vi "Update Graphs_Brass.vi"(0 "Select Graph":T8=enum."Water Temperature (F)", 2 "appended array":refnum<vi>[](array[refnum]), 5 "ERD Graph  Ind 2":T7, 7 "All_Bundled_Data_Brass":T1, 11 "Error In":errorcluster) -> (3 "Dryer Loads":dbl[][](graph), 4 "Washer Loads":u16[][](graph)=[[0, 100, 200, 300, 400]], 6 "Water Temperature":dbl(graph), 8 "Basket Speed":u16(graph), 10 "Pressure":dbl(graph), 12 "ERD 3":dbl(graph), 13 "ERD 2":dbl(graph), 14 "ERD 1":dbl(graph), 15 "Error Out":errorcluster)   [LabVIEW 2016]
doc: "This VI displays (makes visable) the corresponding graph based on user selection, as well as updates the values of the graphs with current data."
uses:
  type defs2/Select _Graph_Brass.ctl
  type defs2/All_Bundled_Data_Brass.ctl
  Laundry Tool 1.0 Support/type defs/Version.ctl
  type defs2/ERD_Always_Show_Brass.ctl
  type defs2/CSV_File_String_Arrays.ctl
  type defs2/Fault Table Array.ctl
  Laundry Tool 1.0 Support/type defs/Fault_Table_Info.ctl
panel:
  # "Software Version"
  # "UI - Critical Version"
  # "UI - Non-Critical"
  # "MC -  Version"
  # "Inverter Version"
  # "Model Setting"
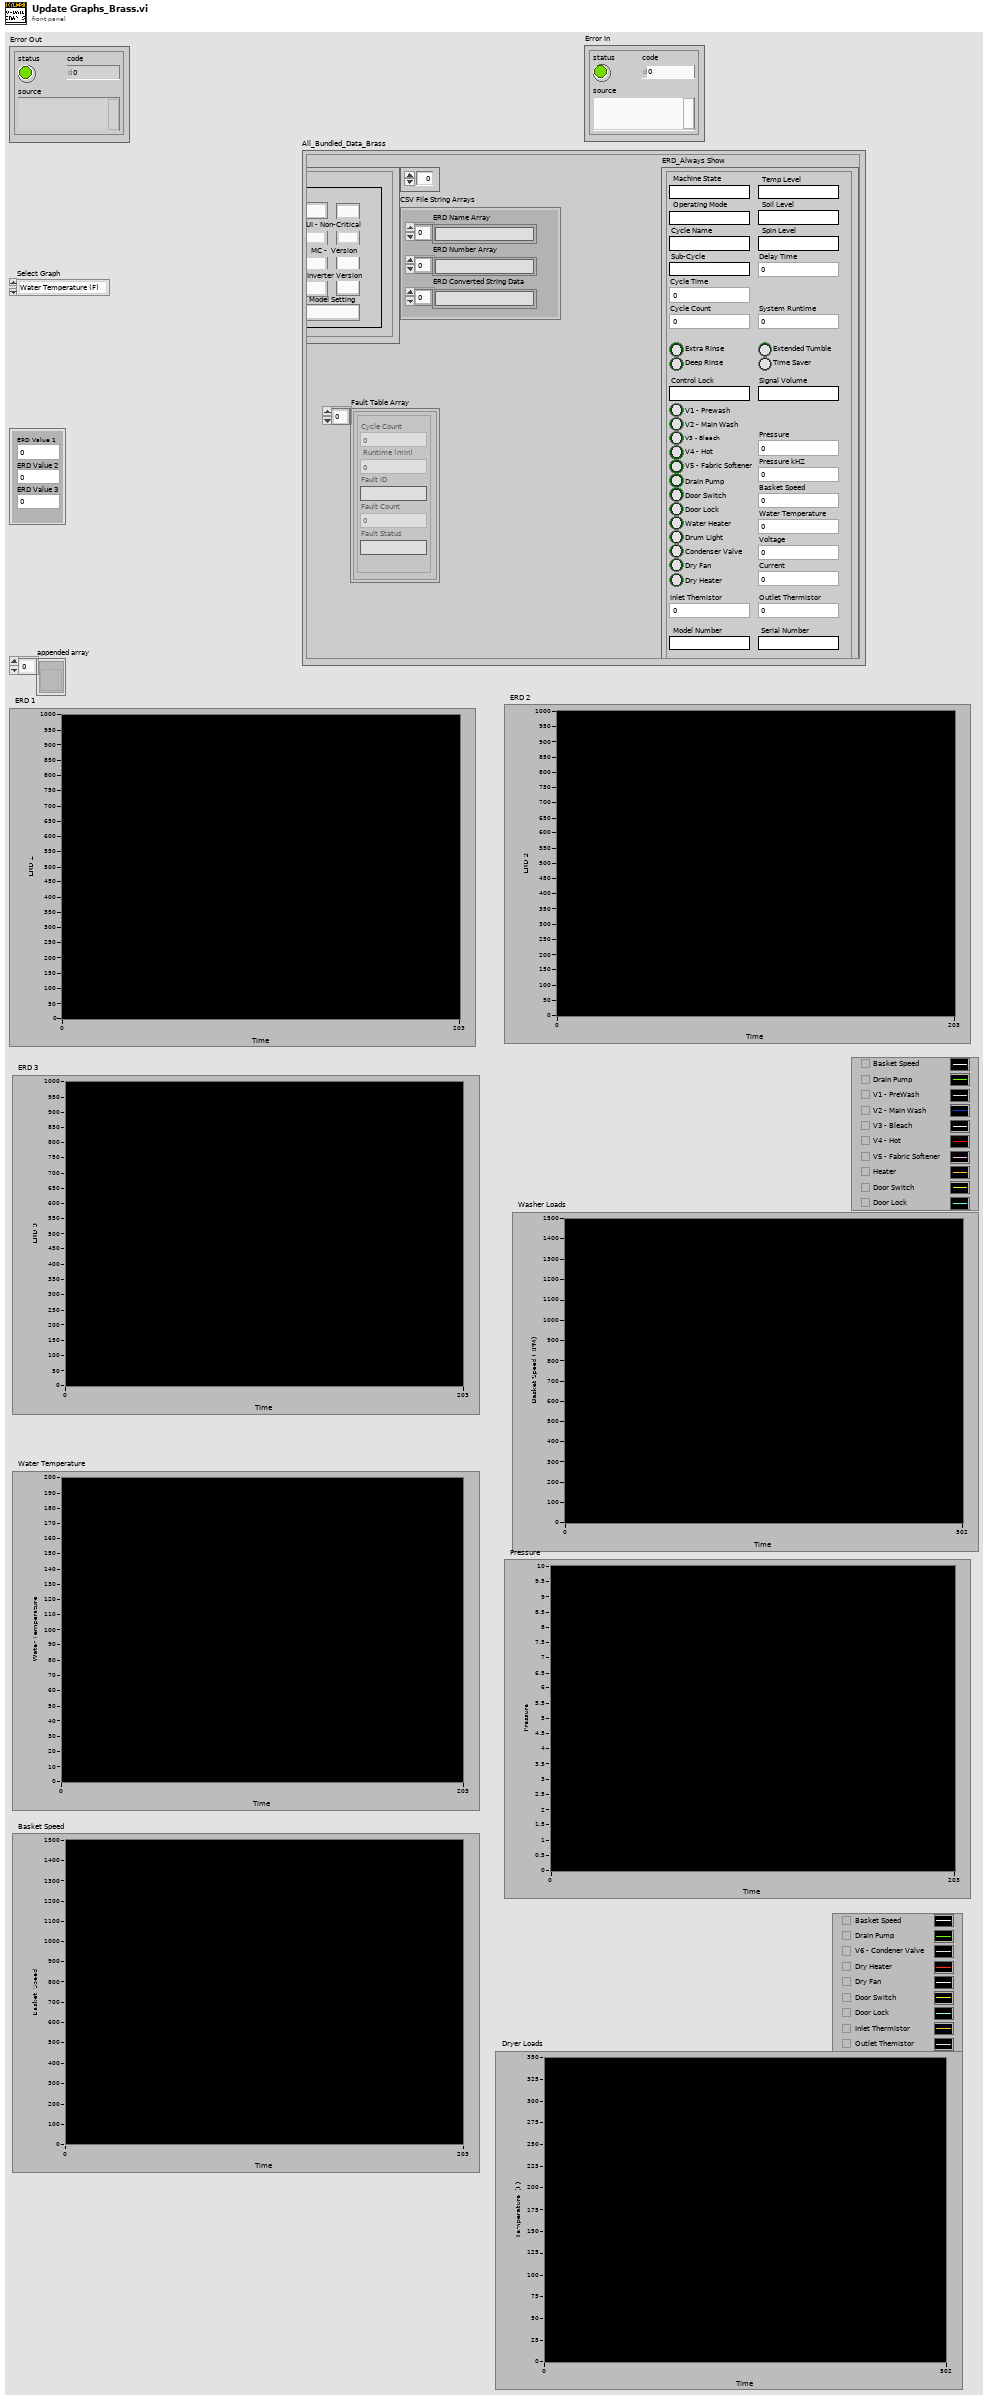
[diagram p1: front panel]
types:
  T1 = typedef "All_Bundled_Data_Brass.ctl" = cluster{"Version":T2, "ERD_Always Show":T3, "Personality Set":u8, "CSV File String Arrays":T4, "Fault Table Array ":T5}
  T2 = typedef "Version.ctl" = cluster{"UI - Critical Major":string, "UI - Critical Minor":string, "UI - Non-Critical Minor":string, "UI - Non-Critical Major":string, "MC Minor":string, "MC Major":string, "Model Setting":string, "Inverter Version  Minor":string, "Inverter Version Major":string}
  T3 = typedef "ERD_Always_Show_Brass.ctl" = cluster{"Machine State":string, "Cycle Count":u32, "Soil Level":string, "Spin Level":string, "Temp Level":string, "Delay Time":u16, "Sub-Cycle":string, "Cycle Name":string, "Model Number":string, "Serial Number":string, "System Runtime":u32, "Cycle Time":u16, "Operating Mode":string, "Deep Rinse":bool, "Extra Rinse":bool, "V1 - Prewash":bool, "V2 - Main Wash":bool, "V3 - Bleach":bool, "V4 - Hot":bool, "Drain Pump":bool, "Door Switch":bool, "Door Lock":bool, "Basket Speed":u16, "Water Temperature":dbl, "Voltage":dbl, "Pressure":dbl, "Water Heater":bool, "Control Lock":string, "Signal Volume":string, "Current":u16, "Pressure kHZ":dbl, "Drum Light":bool, "V5 - Fabric Softener":bool, "Inlet Themistor":dbl, "Outlet Thermistor":dbl, "Condenser Valve":bool, "Dry Fan":bool, "Dry Heater":bool, "Extended Tumble":bool, "Time Saver":bool}
  T4 = typedef "CSV_File_String_Arrays.ctl" = cluster{"ERD Number Array":string[], "ERD Name Array":string[], "ERD Converted String Data":string[]}
  T5 = typedef "Fault Table Array.ctl" = T6[]
  T6 = typedef "Fault_Table_Info.ctl" = cluster{"Cycle Count":u32, " Runtime (min) ":u32, "Fault Status":string, "Fault ID":string, "Fault Count":u16}
  T7 = cluster{"ERD Value 1":dbl, "ERD Value 2":dbl, "ERD Value 3":dbl}
  T8 = typedef "Select _Graph_Brass.ctl" = enum16{"Washer Loads", "Dryer Loads", "ERD 1", "ERD 2", "ERD 3", "Water Temperature (F)", "Basket Speed (RPM)", "Pressure (in H2O)"}
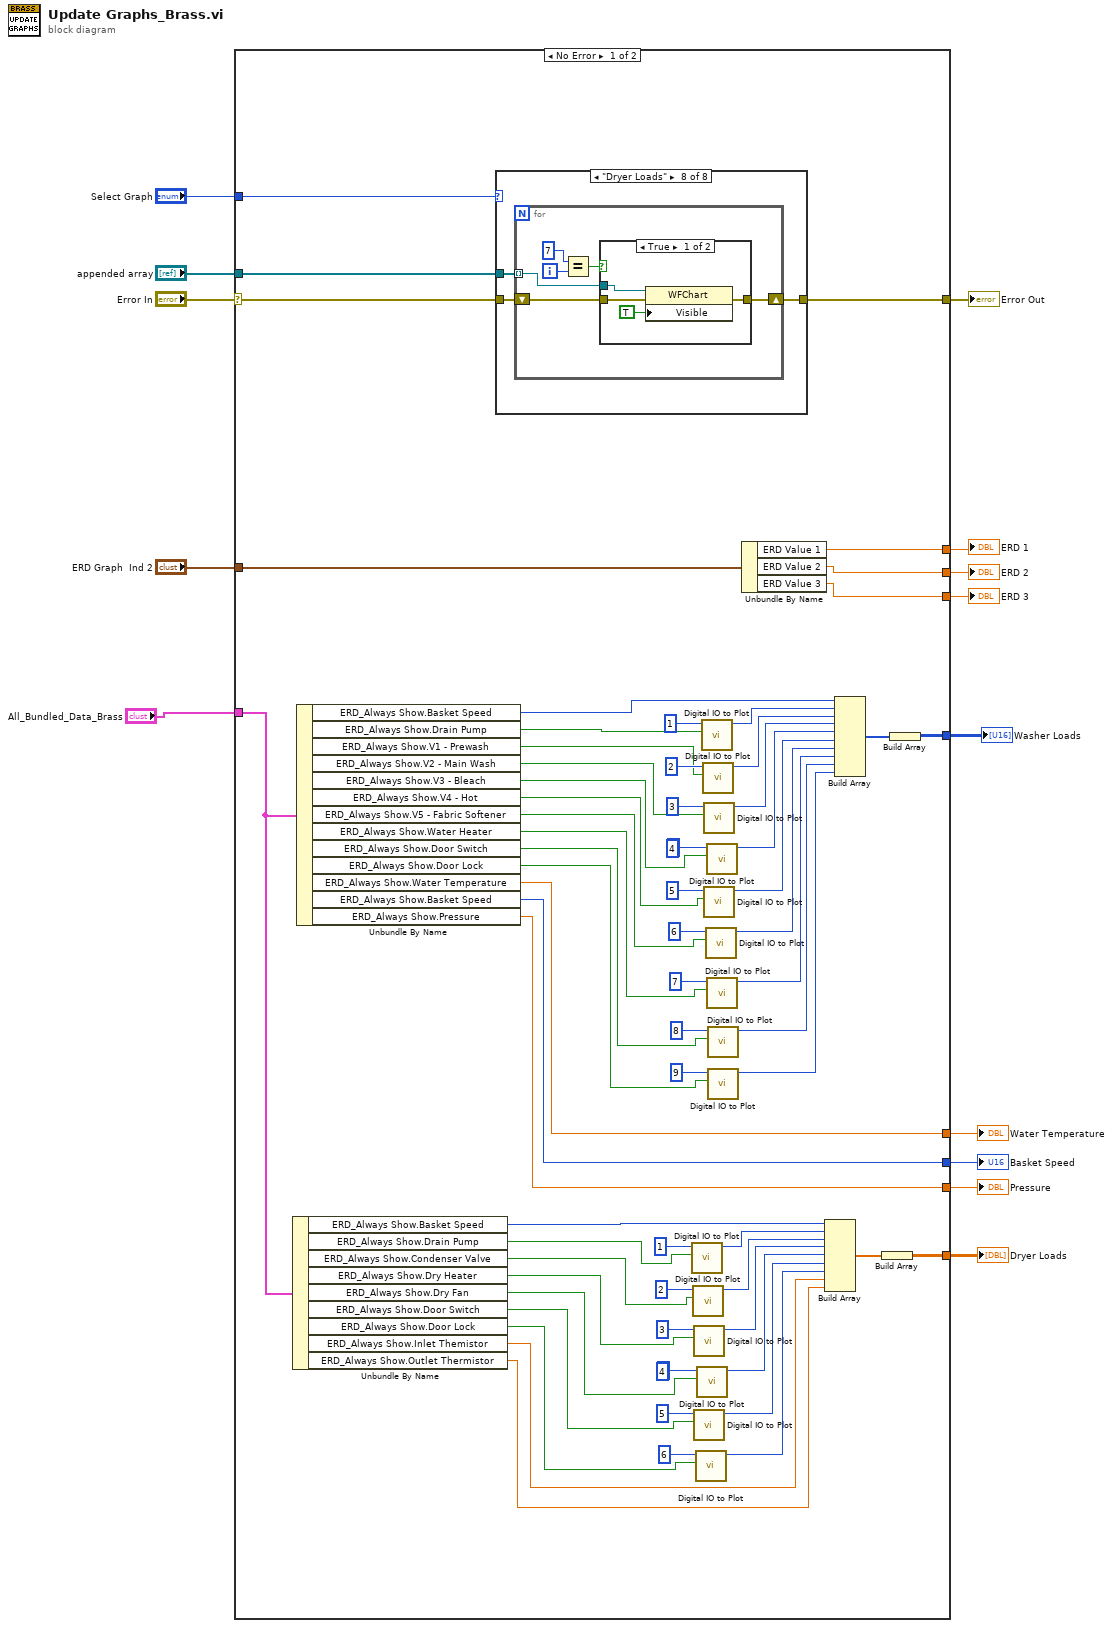
[diagram p0: block diagram]
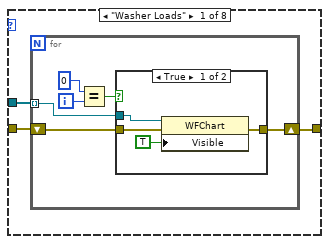
[diagram p2: hidden frame]
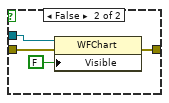
[diagram p3: hidden frame]
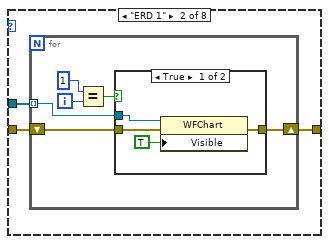
[diagram p4: hidden frame]
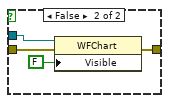
[diagram p5: hidden frame]
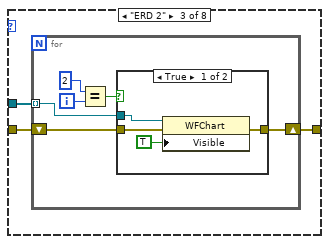
[diagram p6: hidden frame]
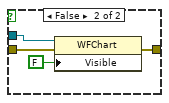
[diagram p7: hidden frame]
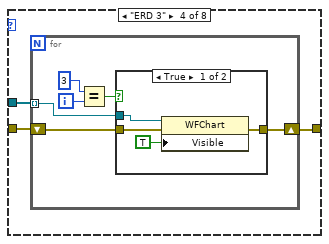
[diagram p8: hidden frame]
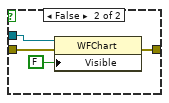
[diagram p9: hidden frame]
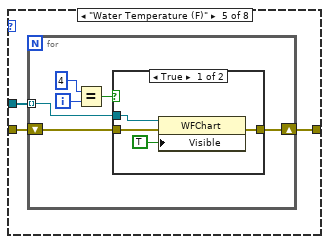
[diagram p10: hidden frame]
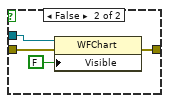
[diagram p11: hidden frame]
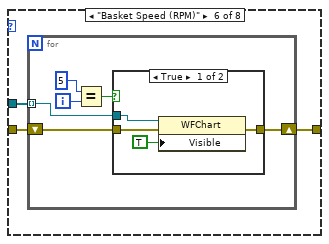
[diagram p12: hidden frame]
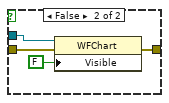
[diagram p13: hidden frame]
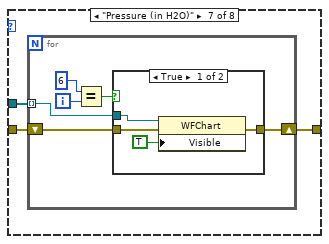
[diagram p14: hidden frame]
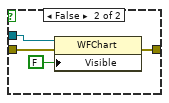
[diagram p15: hidden frame]
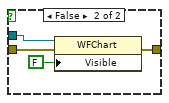
[diagram p16: hidden frame]
diagram:
  n1 = case shown="No Error" "Error In" {
    selector: "Error In" -> [w77 w216]
    tunnel: [w76 w216] -> w13
    tunnel: "appended array" -> [w78 _]
    tunnel: "Select Graph" -> [w79 _]
    tunnel: "ERD Graph  Ind 2" -> [w75 _]
    tunnel: [w74 _] -> w9
    tunnel: [w73 _] -> w8
    tunnel: [w72 _] -> w7
    tunnel: "All_Bundled_Data_Brass" -> [w24 _]
    tunnel: [w69 _] -> w6
    tunnel: [w49 _] -> w4
    tunnel: [w48 _] -> w3
    tunnel: [w47 _] -> w2
    tunnel: [w25 _] -> w1
    frame No Error {
      (unwired) u16 4 ("Multiplier")
      (unwired) u16 4 ("Multiplier")
      n2 = Unbundle By Name(w24) -> ("ERD_Always Show.Basket Speed"=w23:u16, "ERD_Always Show.Drain Pump"=w22:bool, "ERD_Always Show.Condenser Valve"=w21:bool, "ERD_Always Show.Dry Heater"=w20:bool, "ERD_Always Show.Dry Fan"=w19:bool, "ERD_Always Show.Door Switch"=w18:bool, "ERD_Always Show.Door Lock"=w17:bool, "ERD_Always Show.Inlet Themistor"=w16:dbl, "ERD_Always Show.Outlet Thermistor"=w15:dbl)
      n3 = Unbundle By Name(w24) -> ("ERD_Always Show.Basket Speed"=w71:u16, "ERD_Always Show.Drain Pump"=w68:bool, "ERD_Always Show.V1 - Prewash"=w64:bool, "ERD_Always Show.V2 - Main Wash"=w63:bool, "ERD_Always Show.V3 - Bleach"=w46:bool, "ERD_Always Show.V4 - Hot"=w54:bool, "ERD_Always Show.V5 - Fabric Softener"=w44:bool, "ERD_Always Show.Water Heater"=w43:bool, "ERD_Always Show.Door Switch"=w42:bool, "ERD_Always Show.Door Lock"=w40:bool, "ERD_Always Show.Water Temperature"=w49:dbl, "ERD_Always Show.Basket Speed"=w47:u16, "ERD_Always Show.Pressure"=w48:dbl)
      n4 = case shown="\"Dryer Loads\"" w79 {
        tunnel: w78 -> [w80 w98 w116 w131 w150 w167 w184 w201]
        tunnel: w77 -> [w82 w99 w115 w133 w149 w166 w183 w200]
        tunnel: [w81 w97 w114 w132 w148 w165 w182 w199] -> w76
        frame "Washer Loads" {
          n5 = for {
            tunnel: w80 -> [w88] mode=indexing
            shift-right: [w86] -> w81
            shift-left: w82 -> [w87]
            i -> [w85]
            n6 = Equal?(x=0 ("index"), y=w85) -> (x = y?=w83:bool)
            n7 = case shown="True" w83 {
              tunnel: w88 -> [w92 w96]
              tunnel: w87 -> [w90 w94]
              tunnel: [w89 w93] -> w86
              frame True {
                n8 = property class="WFChart"(reference=w92, error in=w90, "Visible"=TRUE) -> (error out=w89:errorcluster)  [unwired: 1 out]
              }
              frame False {
                n9 = property class="WFChart"(reference=w96, error in=w94, "Visible"=FALSE) -> (error out=w93:errorcluster)  [unwired: 1 out]
              }
            }
          }
        }
        frame "ERD 1" {
          n10 = for {
            tunnel: w98 -> [w105] mode=indexing
            shift-right: [w103] -> w97
            shift-left: w99 -> [w104]
            i -> [w102]
            n11 = Equal?(x=1 ("index"), y=w102) -> (x = y?=w100:bool)
            n12 = case shown="True" w100 {
              tunnel: w105 -> [w109 w113]
              tunnel: w104 -> [w107 w111]
              tunnel: [w106 w110] -> w103
              frame True {
                n13 = property class="WFChart"(reference=w109, error in=w107, "Visible"=TRUE) -> (error out=w106:errorcluster)  [unwired: 1 out]
              }
              frame False {
                n14 = property class="WFChart"(reference=w113, error in=w111, "Visible"=FALSE) -> (error out=w110:errorcluster)  [unwired: 1 out]
              }
            }
          }
        }
        frame "ERD 2" {
          n15 = for {
            tunnel: w116 -> [w122] mode=indexing
            shift-right: [w120] -> w114
            shift-left: w115 -> [w121]
            i -> [w119]
            n16 = Equal?(x=2 ("index"), y=w119) -> (x = y?=w117:bool)
            n17 = case shown="True" w117 {
              tunnel: w122 -> [w126 w130]
              tunnel: w121 -> [w124 w128]
              tunnel: [w123 w127] -> w120
              frame True {
                n18 = property class="WFChart"(reference=w126, error in=w124, "Visible"=TRUE) -> (error out=w123:errorcluster)  [unwired: 1 out]
              }
              frame False {
                n19 = property class="WFChart"(reference=w130, error in=w128, "Visible"=FALSE) -> (error out=w127:errorcluster)  [unwired: 1 out]
              }
            }
          }
        }
        frame "ERD 3" {
          n20 = for {
            tunnel: w131 -> [w139] mode=indexing
            shift-right: [w137] -> w132
            shift-left: w133 -> [w138]
            i -> [w136]
            n21 = Equal?(x=3 ("index"), y=w136) -> (x = y?=w134:bool)
            n22 = case shown="True" w134 {
              tunnel: w139 -> [w143 w147]
              tunnel: w138 -> [w141 w145]
              tunnel: [w140 w144] -> w137
              frame True {
                n23 = property class="WFChart"(reference=w143, error in=w141, "Visible"=TRUE) -> (error out=w140:errorcluster)  [unwired: 1 out]
              }
              frame False {
                n24 = property class="WFChart"(reference=w147, error in=w145, "Visible"=FALSE) -> (error out=w144:errorcluster)  [unwired: 1 out]
              }
            }
          }
        }
        frame "Water Temperature (F)" {
          n25 = for {
            tunnel: w150 -> [w156] mode=indexing
            shift-right: [w154] -> w148
            shift-left: w149 -> [w155]
            i -> [w153]
            n26 = Equal?(x=4 ("index"), y=w153) -> (x = y?=w151:bool)
            n27 = case shown="True" w151 {
              tunnel: w156 -> [w160 w164]
              tunnel: w155 -> [w158 w162]
              tunnel: [w157 w161] -> w154
              frame True {
                n28 = property class="WFChart"(reference=w160, error in=w158, "Visible"=TRUE) -> (error out=w157:errorcluster)  [unwired: 1 out]
              }
              frame False {
                n29 = property class="WFChart"(reference=w164, error in=w162, "Visible"=FALSE) -> (error out=w161:errorcluster)  [unwired: 1 out]
              }
            }
          }
        }
        frame "Basket Speed (RPM)" {
          n30 = for {
            tunnel: w167 -> [w173] mode=indexing
            shift-right: [w171] -> w165
            shift-left: w166 -> [w172]
            i -> [w170]
            n31 = Equal?(x=5 ("index"), y=w170) -> (x = y?=w168:bool)
            n32 = case shown="True" w168 {
              tunnel: w173 -> [w177 w181]
              tunnel: w172 -> [w175 w179]
              tunnel: [w174 w178] -> w171
              frame True {
                n33 = property class="WFChart"(reference=w177, error in=w175, "Visible"=TRUE) -> (error out=w174:errorcluster)  [unwired: 1 out]
              }
              frame False {
                n34 = property class="WFChart"(reference=w181, error in=w179, "Visible"=FALSE) -> (error out=w178:errorcluster)  [unwired: 1 out]
              }
            }
          }
        }
        frame "Pressure (in H2O)" {
          n35 = for {
            tunnel: w184 -> [w190] mode=indexing
            shift-right: [w188] -> w182
            shift-left: w183 -> [w189]
            i -> [w187]
            n36 = Equal?(x=6 ("index"), y=w187) -> (x = y?=w185:bool)
            n37 = case shown="True" w185 {
              tunnel: w190 -> [w194 w198]
              tunnel: w189 -> [w192 w196]
              tunnel: [w191 w195] -> w188
              frame True {
                n38 = property class="WFChart"(reference=w194, error in=w192, "Visible"=TRUE) -> (error out=w191:errorcluster)  [unwired: 1 out]
              }
              frame False {
                n39 = property class="WFChart"(reference=w198, error in=w196, "Visible"=FALSE) -> (error out=w195:errorcluster)  [unwired: 1 out]
              }
            }
          }
        }
        frame "Dryer Loads" {
          n40 = for {
            tunnel: w201 -> [w207] mode=indexing
            shift-right: [w205] -> w199
            shift-left: w200 -> [w206]
            i -> [w204]
            n41 = Equal?(x=7 ("index"), y=w204) -> (x = y?=w202:bool)
            n42 = case shown="True" w202 {
              tunnel: w207 -> [w211 w215]
              tunnel: w206 -> [w209 w213]
              tunnel: [w208 w212] -> w205
              frame True {
                n43 = property class="WFChart"(reference=w211, error in=w209, "Visible"=TRUE) -> (error out=w208:errorcluster)  [unwired: 1 out]
              }
              frame False {
                n44 = property class="WFChart"(reference=w215, error in=w213, "Visible"=FALSE) -> (error out=w212:errorcluster)  [unwired: 1 out]
              }
            }
          }
        }
      }
      n45 = call "Digital IO to Plot.vi"("Boolean Value"=w22, "Multiplier"=u16 1) -> ("Output"=w34:u16)  [unwired: 9 in]
      n46 = call "Digital IO to Plot.vi"("Boolean Value"=w21, "Multiplier"=u16 2) -> ("Output"=w33:u16)  [unwired: 9 in]
      n47 = call "Digital IO to Plot.vi"("Boolean Value"=w20, "Multiplier"=u16 3) -> ("Output"=w32:u16)  [unwired: 9 in]
      n48 = call "Digital IO to Plot.vi"("Boolean Value"=w18, "Multiplier"=u16 5) -> ("Output"=w28:u16)  [unwired: 9 in]
      n49 = call "Digital IO to Plot.vi"("Boolean Value"=w17, "Multiplier"=u16 6) -> ("Output"=w27:u16)  [unwired: 9 in]
      n50 = call "Digital IO to Plot.vi"("Boolean Value"=w19, "Multiplier"=u16 4) -> ("Output"=w26:u16)  [unwired: 9 in]
      n51 = call "Digital IO to Plot.vi"("Boolean Value"=w68, "Multiplier"=u16 1) -> ("Output"=w62:u16)  [unwired: 9 in]
      n52 = call "Digital IO to Plot.vi"("Boolean Value"=w64, "Multiplier"=u16 2) -> ("Output"=w61:u16)  [unwired: 9 in]
      n53 = call "Digital IO to Plot.vi"("Boolean Value"=w63, "Multiplier"=u16 3) -> ("Output"=w60:u16)  [unwired: 9 in]
      n54 = call "Digital IO to Plot.vi"("Boolean Value"=w54, "Multiplier"=u16 5) -> ("Output"=w56:u16)  [unwired: 9 in]
      n55 = call "Digital IO to Plot.vi"("Boolean Value"=w44, "Multiplier"=u16 6) -> ("Output"=w55:u16)  [unwired: 9 in]
      n56 = call "Digital IO to Plot.vi"("Boolean Value"=w46, "Multiplier"=u16 4) -> ("Output"=w45:u16)  [unwired: 9 in]
      n57 = call "Digital IO to Plot.vi"("Boolean Value"=w43, "Multiplier"=u16 7) -> ("Output"=w52:u16)  [unwired: 9 in]
      n58 = call "Digital IO to Plot.vi"("Boolean Value"=w42, "Multiplier"=u16 8) -> ("Output"=w51:u16)  [unwired: 9 in]
      n59 = call "Digital IO to Plot.vi"("Boolean Value"=w40, "Multiplier"=u16 9) -> ("Output"=w39:u16)  [unwired: 9 in]
      n60 = Unbundle By Name(w75) -> ("ERD Value 1"=w74:dbl, "ERD Value 2"=w73:dbl, "ERD Value 3"=w72:dbl)
      n61 = Build Array(w23, w34, w33, w32, w26, w28, w27, w16, w15) -> (w38:dbl[])
      n62 = Build Array(w71, w62, w61, w60, w45, w56, w55, w52, w51, w39) -> (w70:u16[])
      n63 = Build Array(w38) -> (w25:dbl[][])
      n64 = Build Array(w70) -> (w69:u16[][])
    }
    frame Error {
    }
  }
  "Error Out" <- w13
  "ERD 1" <- w9
  "ERD 2" <- w8
  "ERD 3" <- w7
  "Washer Loads" <- w6
  "Water Temperature" <- w4
  "Pressure" <- w3
  "Basket Speed" <- w2
  "Dryer Loads" <- w1
